vi "New File.vi"(8 "Error In":errorcluster, 11 "Text File in":refnum<class "Text File.lvclass">) -> (0 "error out":errorcluster, 3 "Text File out":refnum<class "Text File.lvclass">)   [LabVIEW 2019, in "TSC Event Logger.lvlib" / "Text File.lvclass"]
doc: "Create a new log sink of text file type.\n\n<b>Code Developed By:</b>\nTechnology Service Corporation\nBloomington, IN 47403\nwww.tsc.com/atcs\n\nDeveloper:\nDaniel Coons"
uses:
  Text File.lvclass
  Text File.lvclass/Text File.ctl
  Log Sinks.lvclass
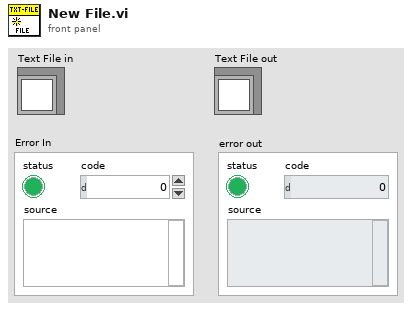
[diagram p1: front panel]
types:
  T1 = enum16{"open", "replace", "create", "open or create", "replace or create", "replace or create with confirmation"}
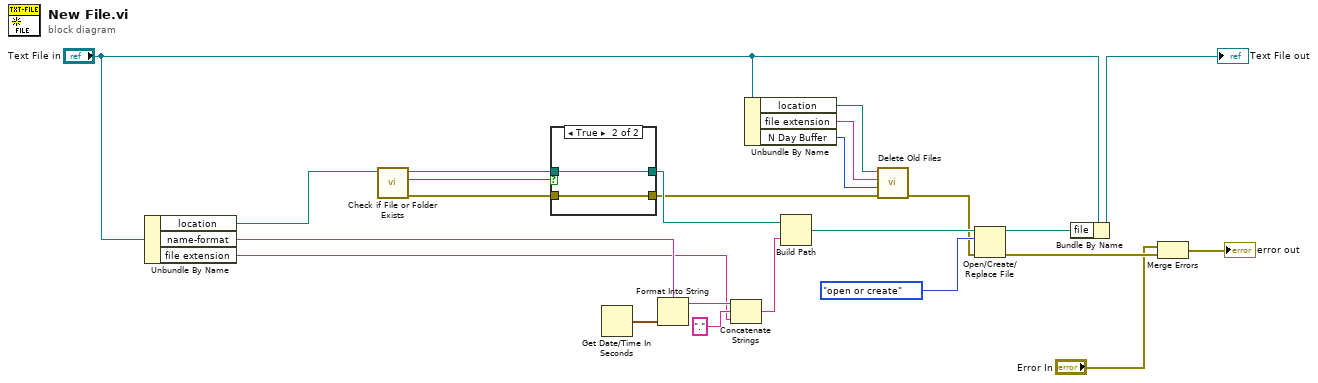
[diagram p0: block diagram]
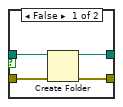
[diagram p2: hidden frame]
diagram:
  n1 = Unbundle By Name("Text File in") -> ("location"=w10:path, "name-format"=w16:string, "file extension"=w8:string)
  n2 = call <vilib>:"Check if File or Folder Exists.vi"("path"=w10) -> ("error out"=w9:errorcluster, "file or folder exists?"=w11:bool, "dup path"=w12:path)  [unwired: 8 in]
  n3 = case shown="True" w11 {
    tunnel: w12 -> [w28 w30]
    tunnel: [w27 w30] -> w7
    tunnel: w9 -> [w26 w29]
    tunnel: [w25 w29] -> w6
    frame False {
      n4 = Create Folder(path (use dialog)=w28, error in=w26) -> (created path=w27:path, error out=w25:errorcluster)  [unwired: 1 in, 1 out]
    }
    frame True {
    }
  }
  n5 = Get Date/Time In Seconds() -> (seconds since 1Jan1904=w23:timestamp)
  n6 = Format Into String(format string=w16, w23) -> (resulting string=w24:string)  [unwired: 2 in, 1 out]
  n7 = Concatenate Strings(w24, "." ("string"), w8) -> (w22:string)
  n8 = Unbundle By Name("Text File in") -> ("location"=w1:path, "file extension"=w2:string, "N Day Buffer"=w3:u32)
  n9 = Build Path(base path=w7, name or relative path=w22) -> (appended path=w13:path)
  n10 = call "Delete Old Files.vi"("error in (no error)"=w6, "N Day Buffer"=w3, "file extension"=w2, "location"=w1) -> ("error out"=w5:errorcluster)  [unwired: 7 in]
  n11 = Open/Create/Replace File(file path (use dialog)=w13, error in=w5, operation (0:open)=T1."open or create") -> (refnum out=w19:refnum<file>, error out=w20:errorcluster)  [unwired: 3 in, 1 out]
  n12 = Bundle By Name(cluster="Text File in", "file"=w19) -> (→"Text File out":refnum<class "Text File.lvclass">)
  n13 = Merge Errors("Error In", w20) -> (→"error out":errorcluster)
